vi "WPI_AccumulatorOffset.vi"(8 "error in (no error)":errorcluster, 9 "Offset In":i32, 10 "Action":enum16{"read", "write"}(ring), 11 "AIDeviceRef":T1={"DevStatus"={"status"=FALSE, "code"=0, "source"=""}, "Analog Channel"=enum."AI 1"}) -> (0 "error out":errorcluster, 1 "Offset Out":i32, 3 "AIDeviceRef":T1={"DevStatus"={"status"=FALSE, "code"=0, "source"=""}, "Analog Channel"=enum."AI 1"})   [LabVIEW 2017]
doc: "This software is licensed. Open the labview\\readme\\WPI Robotics Library Open Source License.txt file for more information."
uses:
  <vilib>/Rock Robotics/WPI/AnalogChannel/WPI_AnalogChannelDevRef.ctl
  <vilib>/Rock Robotics/SystemInterfaces/AI/FPGA_AIChannel.ctl
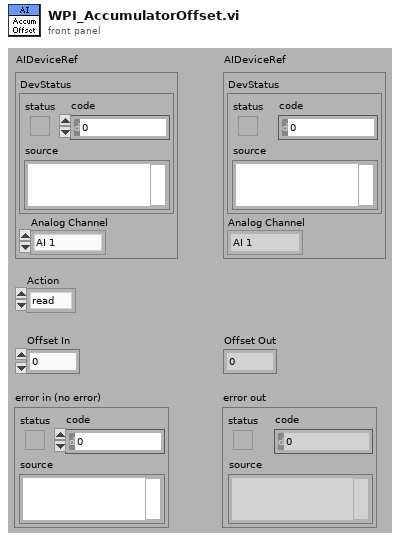
[diagram p1: front panel]
types:
  T1 = typedef "WPI_AnalogChannelDevRef.ctl" = cluster{"DevStatus":errorcluster, "Analog Channel":T2}
  T2 = typedef "FPGA_AIChannel.ctl" = enum8{"AI 0", "AI 1", "AI 2", "AI 3", "AI MXP 0", "AI MXP 1", "AI MXP 2", "AI MXP 3", "Invalid"}
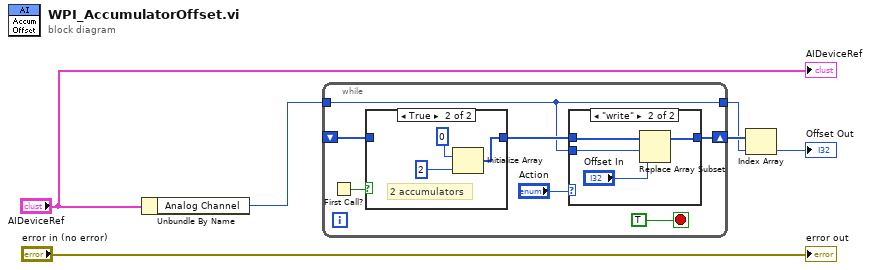
[diagram p0: block diagram]
diagram:
  n1 = Unbundle By Name("AIDeviceRef") -> ("Analog Channel"=w1:T2)
  n2 = while {
    shift-right: [w12] -> w3
    shift-left: _ -> [w9]
    tunnel: w1 -> [w7]
    tunnel: [w7] -> w2
    stop <- TRUE stop-if-true
    n3 = First Call?() -> (First Call?: T/F=w10:bool)
    n4 = case shown="True" w10 {
      tunnel: w9 -> [w14 _]
      tunnel: [w14 w17] -> w8
      frame False {
      }
      frame True {
        # "2 accumulators"
        n5 = Initialize Array(0 ("element"), 2 ("dimension size")) -> (w17:i32[])
      }
    }
    n6 = case shown="\"write\"" "Action" {
      tunnel: [w18 w21] -> w12
      tunnel: w8 -> [w18 w22]
      tunnel: w7 -> [_ w20]
      frame "read", Default {
      }
      frame "write" {
        n7 = Replace Array Subset(array=w22, new element="Offset In", index=w20) -> (w21:i32[])
      }
    }
  }
  n8 = Index Array(array=w3, index=w2) -> (element=→"Offset Out":i32)
  "AIDeviceRef" <- "AIDeviceRef"
  "error out" <- "error in (no error)"
